vi "HEWH Calc Convert Pressure.vi"(8 "All Data":dbl[](array[numeric]) format="%.4f") -> (0 "output array":dbl[](array[numeric]))   [LabVIEW 2012]
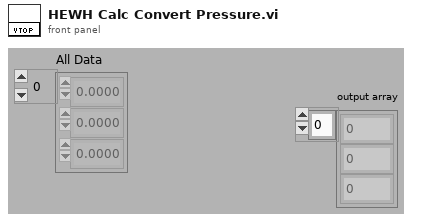
[diagram p1: front panel]
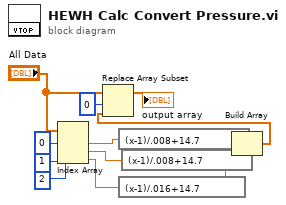
[diagram p0: block diagram]
diagram:
  n1 = Index Array(array="All Data", index #1=0 ("index"), index #2=1 ("index"), index #3=2 ("index")) -> (element #1=w8:dbl, element #2=w6:dbl, element #3=w7:dbl)
  n2 = expression code="(x-1)/.008+14.7"(w8) -> (w3:dbl)
  n3 = expression code="(x-1)/.016+14.7"(w7) -> (w5:dbl)
  n4 = expression code="(x-1)/.008+14.7"(w6) -> (w4:dbl)
  n5 = Build Array(w3, w4, w5) -> (w2:dbl[])
  n6 = Replace Array Subset(array="All Data", new element=w2, index=0) -> (→"output array":dbl[])
